vi "Test_monitorCommand_abort.vi"(8 "error in (no error)":errorcluster, 11 "command_abort_Ctl":T1) -> (0 "error out":errorcluster, 2 "function return":i32, 3 "command_abort_Ctl out":T1)   [LabVIEW 2016, in "SALLV_Test.lvlib"]
doc: "int Test_shm_monitorCommand_abortLV(Test_command_abortLV *command_abort_Ctl );"
uses:
  SALLV_Test.lvlib
  DataTypes/command_abort.ctl
  SALLV_Test.so
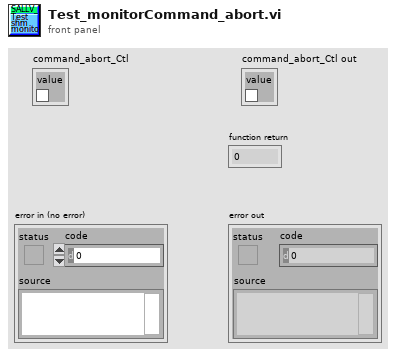
[diagram p1: front panel]
types:
  T1 = typedef "SALLV_Test.lvlib/command_abort.ctl" = cluster{"value":bool}
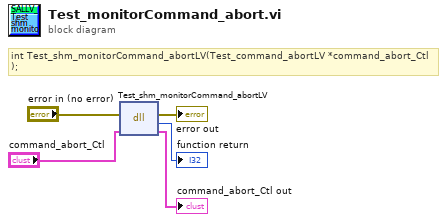
[diagram p0: block diagram]
diagram:
  # "int Test_shm_monitorCommand_abortLV(Test_command_abortLV *command_abort_Ctl );"
  n1 = dll-call lib="home/ccontaxis/Code/SALLV_Test/SALLV_Test.*" fn="Test_shm_monitorCommand_abortLV"(error in="error in (no error)", "command_abort_Ctl"="command_abort_Ctl") -> (error out=→"error out":errorcluster, →"function return":i32, "command_abort_Ctl"=→"command_abort_Ctl out":T1)  [unwired: 2 in, 1 out]
